vi "FL_Filter_data_for_online_display.vi"(2 "Input cluster of SG coefficients":T1, 3 "Input data":cluster{"X1":dbl, "Y1":dbl, "X2":dbl, "Y2":dbl}, 4 "Filter type":u16(ring)=5 items=["None", "Kalman 0.50", "Kalman 0.30", "Kalman 0.12", "Savitzky-Golay 3/5", "Savitzky-Golay 3/11", "Savitzky-Golay 3/31"], 5 "Data filtered on previous step":cluster{"X1":dbl, "Y1":dbl, "X2":dbl, "Y2":dbl}) -> (1 "Output data":cluster{"X1":dbl, "Y1":dbl, "X2":dbl, "Y2":dbl})   [LabVIEW 2018]
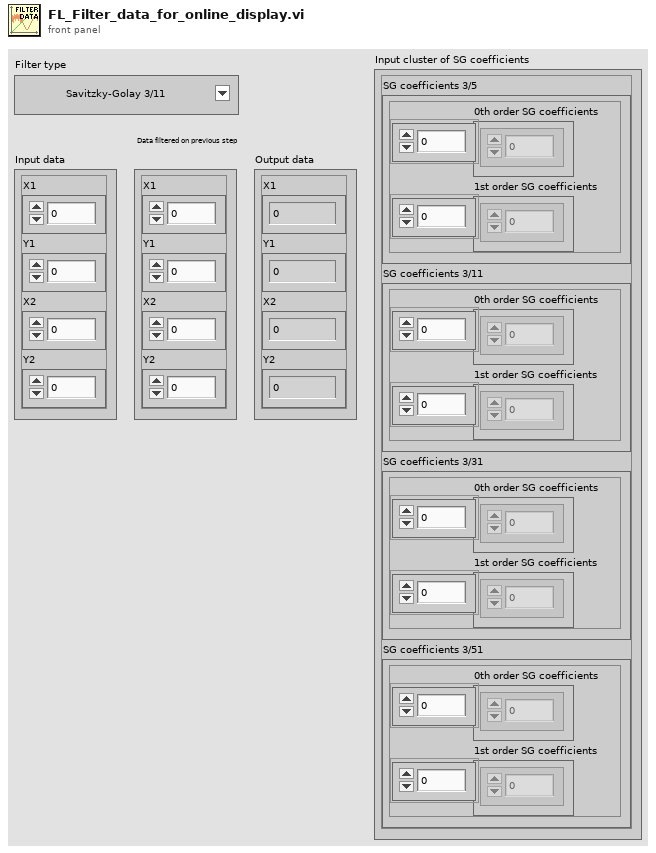
[diagram p1: front panel]
types:
  T1 = cluster{"SG coefficients 3/5":cluster{"0th order SG coefficients":dbl[], "1st order SG coefficients":dbl[]}, "SG coefficients 3/11":cluster{"0th order SG coefficients":dbl[], "1st order SG coefficients":dbl[]}, "SG coefficients 3/31":cluster{"0th order SG coefficients":dbl[], "1st order SG coefficients":dbl[]}, "SG coefficients 3/51":cluster{"0th order SG coefficients":dbl[], "1st order SG coefficients":dbl[]}}
  T2 = cluster{"[0]":dbl, "[1]":dbl, "[2]":dbl, "[3]":dbl}
  T3 = cluster{"0th order SG coefficients":dbl[], "1st order SG coefficients":dbl[]}
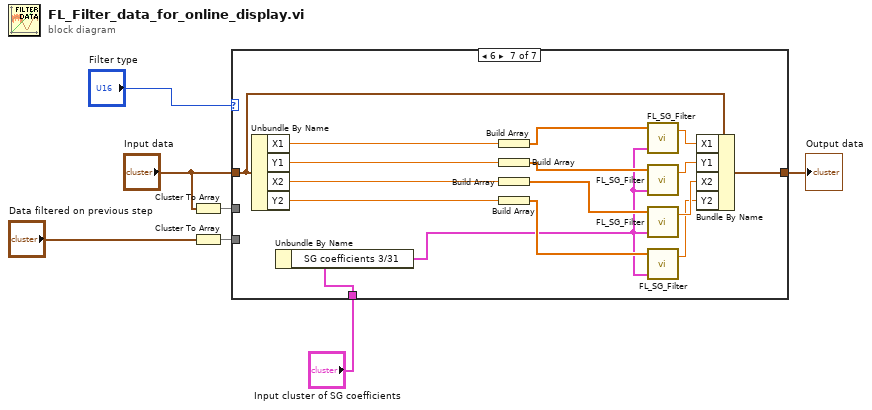
[diagram p0: block diagram]
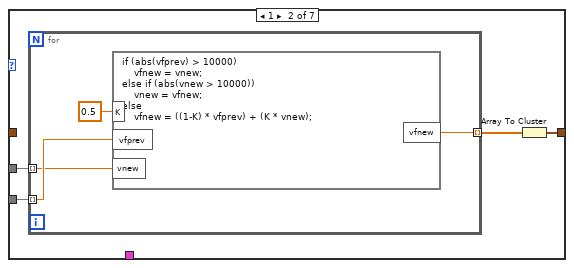
[diagram p3: hidden frame]
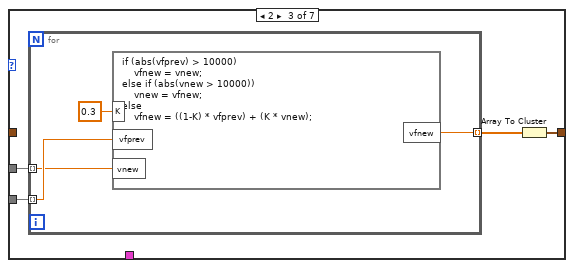
[diagram p4: hidden frame]
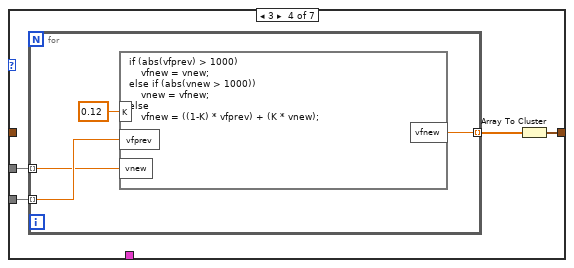
[diagram p5: hidden frame]
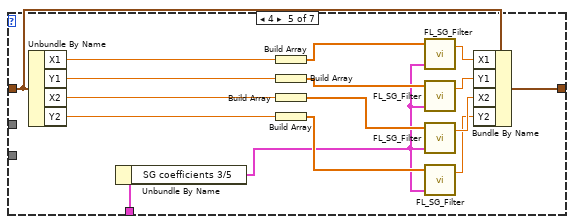
[diagram p6: hidden frame]
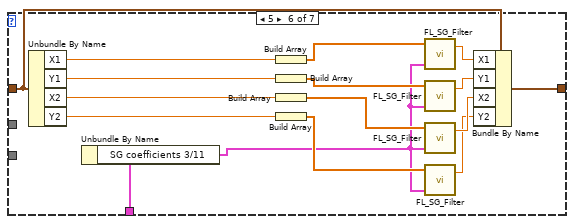
[diagram p7: hidden frame]
diagram:
  n1 = Cluster To Array(cluster="Input data") -> (array=w4:dbl[])
  n2 = Cluster To Array(cluster="Data filtered on previous step") -> (array=w6:dbl[])
  n3 = case shown="6" "Filter type" {
    tunnel: w6 -> [_ w12 w20 w28 _ _ _]
    tunnel: [w8 w10 w18 w26 w35 w51 w67] -> w5
    tunnel: w4 -> [_ w9 w17 w25 _ _ _]
    tunnel: "Input data" -> [w8 _ _ _ w40 w56 w72]
    tunnel: "Input cluster of SG coefficients" -> [_ _ _ _ w34 w50 w66]
    frame 0, Default {
    }
    frame 1 {
      n4 = for {
        tunnel: w9 -> [w15] mode=indexing
        tunnel: w12 -> [w16] mode=indexing
        tunnel: [w14] -> w11 mode=indexing
        n5 = formula code="if (abs(vfprev) > 10000)\n    vfnew = vnew;\nelse if (abs(vnew > 10000))\n    vnew = vfnew;\nelse\n    vfnew = ((1-K) * vfprev) + (K * vnew);"("K"=0.5 ("input variable"), "vfprev"=w16, "vnew"=w15) -> ("vfnew"=w14:dbl)
      }
      n6 = Array To Cluster(array=w11) -> (cluster=w10:T2)
    }
    frame 2 {
      n7 = for {
        tunnel: w17 -> [w23] mode=indexing
        tunnel: w20 -> [w24] mode=indexing
        tunnel: [w22] -> w19 mode=indexing
        n8 = formula code="if (abs(vfprev) > 10000)\n    vfnew = vnew;\nelse if (abs(vnew > 10000))\n    vnew = vfnew;\nelse\n    vfnew = ((1-K) * vfprev) + (K * vnew);"("K"=0.3 ("input variable"), "vfprev"=w24, "vnew"=w23) -> ("vfnew"=w22:dbl)
      }
      n9 = Array To Cluster(array=w19) -> (cluster=w18:T2)
    }
    frame 3 {
      n10 = for {
        tunnel: w25 -> [w31] mode=indexing
        tunnel: w28 -> [w32] mode=indexing
        tunnel: [w30] -> w27 mode=indexing
        n11 = formula code="if (abs(vfprev) > 1000)\n    vfnew = vnew;\nelse if (abs(vnew > 1000))\n    vnew = vfnew;\nelse\n    vfnew = ((1-K) * vfprev) + (K * vnew);"("K"=0.12 ("input variable"), "vfprev"=w32, "vnew"=w31) -> ("vfnew"=w30:dbl)
      }
      n12 = Array To Cluster(array=w27) -> (cluster=w26:T2)
    }
    frame 4 {
      n13 = Unbundle By Name(w40) -> ("X1"=w47:dbl, "Y1"=w45:dbl, "X2"=w44:dbl, "Y2"=w43:dbl)
      n14 = Unbundle By Name(w34) -> ("SG coefficients 3/5"=w33:T3)
      n15 = Build Array(w47) -> (w48:dbl[])
      n16 = Build Array(w45) -> (w46:dbl[])
      n17 = Build Array(w44) -> (w42:dbl[])
      n18 = Build Array(w43) -> (w41:dbl[])
      n19 = call "FL_SG_Filter.vi"("SG coefficients"=w33, "Input array of data"=w48) -> ("Filtered data, 0 order"=w39:dbl)  [unwired: 2 in]
      n20 = call "FL_SG_Filter.vi"("SG coefficients"=w33, "Input array of data"=w46) -> ("Filtered data, 0 order"=w38:dbl)  [unwired: 2 in]
      n21 = call "FL_SG_Filter.vi"("SG coefficients"=w33, "Input array of data"=w42) -> ("Filtered data, 0 order"=w37:dbl)  [unwired: 2 in]
      n22 = call "FL_SG_Filter.vi"("SG coefficients"=w33, "Input array of data"=w41) -> ("Filtered data, 0 order"=w36:dbl)  [unwired: 2 in]
      n23 = Bundle By Name(cluster=w40, "X1"=w39, "Y1"=w38, "X2"=w37, "Y2"=w36) -> (w35:cluster{"X1":dbl, "Y1":dbl, "X2":dbl, "Y2":dbl})
    }
    frame 5 {
      n24 = Unbundle By Name(w56) -> ("X1"=w63:dbl, "Y1"=w61:dbl, "X2"=w60:dbl, "Y2"=w59:dbl)
      n25 = Unbundle By Name(w50) -> ("SG coefficients 3/11"=w49:T3)
      n26 = Build Array(w63) -> (w64:dbl[])
      n27 = Build Array(w61) -> (w62:dbl[])
      n28 = Build Array(w60) -> (w58:dbl[])
      n29 = Build Array(w59) -> (w57:dbl[])
      n30 = call "FL_SG_Filter.vi"("SG coefficients"=w49, "Input array of data"=w64) -> ("Filtered data, 0 order"=w55:dbl)  [unwired: 2 in]
      n31 = call "FL_SG_Filter.vi"("SG coefficients"=w49, "Input array of data"=w62) -> ("Filtered data, 0 order"=w54:dbl)  [unwired: 2 in]
      n32 = call "FL_SG_Filter.vi"("SG coefficients"=w49, "Input array of data"=w58) -> ("Filtered data, 0 order"=w53:dbl)  [unwired: 2 in]
      n33 = call "FL_SG_Filter.vi"("SG coefficients"=w49, "Input array of data"=w57) -> ("Filtered data, 0 order"=w52:dbl)  [unwired: 2 in]
      n34 = Bundle By Name(cluster=w56, "X1"=w55, "Y1"=w54, "X2"=w53, "Y2"=w52) -> (w51:cluster{"X1":dbl, "Y1":dbl, "X2":dbl, "Y2":dbl})
    }
    frame 6 {
      n35 = Unbundle By Name(w72) -> ("X1"=w79:dbl, "Y1"=w77:dbl, "X2"=w76:dbl, "Y2"=w75:dbl)
      n36 = Unbundle By Name(w66) -> ("SG coefficients 3/31"=w65:T3)
      n37 = Build Array(w79) -> (w80:dbl[])
      n38 = Build Array(w77) -> (w78:dbl[])
      n39 = Build Array(w76) -> (w74:dbl[])
      n40 = Build Array(w75) -> (w73:dbl[])
      n41 = call "FL_SG_Filter.vi"("SG coefficients"=w65, "Input array of data"=w80) -> ("Filtered data, 0 order"=w71:dbl)  [unwired: 2 in]
      n42 = call "FL_SG_Filter.vi"("SG coefficients"=w65, "Input array of data"=w78) -> ("Filtered data, 0 order"=w70:dbl)  [unwired: 2 in]
      n43 = call "FL_SG_Filter.vi"("SG coefficients"=w65, "Input array of data"=w74) -> ("Filtered data, 0 order"=w69:dbl)  [unwired: 2 in]
      n44 = call "FL_SG_Filter.vi"("SG coefficients"=w65, "Input array of data"=w73) -> ("Filtered data, 0 order"=w68:dbl)  [unwired: 2 in]
      n45 = Bundle By Name(cluster=w72, "X1"=w71, "Y1"=w70, "X2"=w69, "Y2"=w68) -> (w67:cluster{"X1":dbl, "Y1":dbl, "X2":dbl, "Y2":dbl})
    }
  }
  "Output data" <- w5
